vi "Data to CSV Line.vi"(8 "error in (no error)":errorcluster, 10 "Elapsed Time":string, 11 "Array":waveform(dbl)[](array[waveform])) -> (0 "error out":errorcluster, 2 "Spreadsheet String":string[](array[string]))   [LabVIEW 2021, in "CSV Log.lvlib"]
uses:
  CSV Log.lvlib
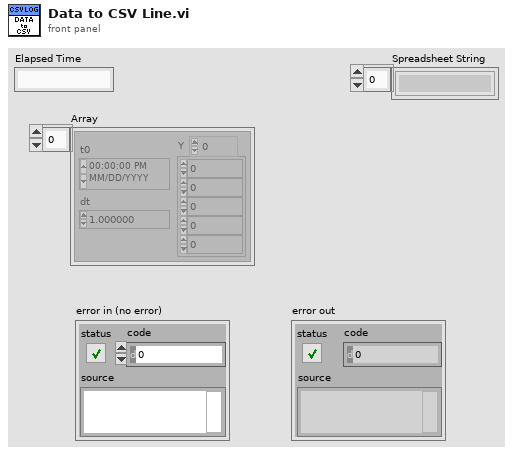
[diagram p1: front panel]
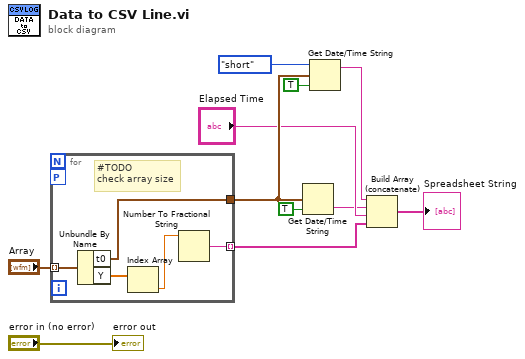
[diagram p0: block diagram]
diagram:
  n1 = for {
    tunnel: "Array" -> [w16] mode=indexing
    tunnel: [w13] -> w6 mode=indexing
    tunnel: [w12] -> w5
    workers-P: _ -> [_]
    # "#TODO\ncheck array size"
    n2 = Unbundle By Name(w16) -> ("t0"=w12:timestamp, "Y"=w15:dbl[])
    n3 = Index Array(array=w15) -> (element=w14:dbl)  [unwired: 1 in]
    n4 = Number To Fractional String(number=w14) -> (F-format string=w13:string)  [unwired: 3 in]
  }
  n5 = Get Date/Time String(seconds (now)=w5, want seconds? (F)=TRUE) -> (time string=w2:string)  [unwired: 1 in, 1 out]
  n6 = Get Date/Time String(date format (0)=enum16{"short", "long", "abbreviated"}."short", seconds (now)=w5, want seconds? (F)=TRUE) -> (date string=w7:string)  [unwired: 1 out]
  n7 = Build Array (concatenate)(w7, w2, "Elapsed Time", w6) -> (→"Spreadsheet String":string[])
  "error out" <- "error in (no error)"
